vi "test.vi"() -> ()   [LabVIEW 2016]
uses:
  <vilib>/Platform/TimedLoop/XDataNode/timing_clust.ctl
  <vilib>/Platform/TimedLoop/XDataNode/nitl_modes.ctl
  <vilib>/Platform/TimedLoop/XDataNode/wakeup.ctl
  <vilib>/FPGAPlugInAG/roboRIO/niLvFpga_Open_roboRIO.vi
  <vilib>/rvi/interface/common/dynamic/niFpgaDynamicAddResources.vi
  <vilib>/FPGAPlugInAG/Dynamic/niLvFpga_Reset_Dynamic.vi
  <vilib>/FPGAPlugInAG/Dynamic/niLvFpga_Run_Dynamic.vi
  <vilib>/Utility/error.llb/Error Cluster From Error Code.vi
  <vilib>/rvi/errors/niLvFpgaAdjustHostInterfaceError.vi
  <vilib>/FPGAPlugInAG/Dynamic/niLvFpga_Abort_Dynamic.vi
  <vilib>/FPGAPlugInAG/Dynamic/niLvFpga_Close_Dynamic.vi
  <vilib>/rvi/interface/nirviOpenFPGA/nirviOpenFPGA.xnode
  FPGA Bitfiles/AutoBikeProject_FPGATarget_AutoBikeFPGA_EwzLm8KNttI.lvbitx
  <vilib>/rvi/interface/nirviMethod/nirviMethod.xnode
  <vilib>/platform/TimedLoop/XDataNode/XDataNode.xnode
  <vilib>/rvi/interface/nirviReadWriteControl/nirviReadWriteControl.xnode
  <vilib>/rvi/interface/nirviCloseFPGA/nirviCloseFPGA.xnode
  NiFpgaLv.dll
  <vilib>/rvi/interface/Simulation/niFpgaSimulationCallBeginRW.vi
  <vilib>/Platform/TimedLoop/XDataNode/XDNodeRunTimeDep.lvlib
panel:
  out "x+y":i32
  out "Finished Late? [i-1]":bool
  out "error out":errorcluster
  in  "Boolean":bool
  out "Current velocity":sgl(graph)
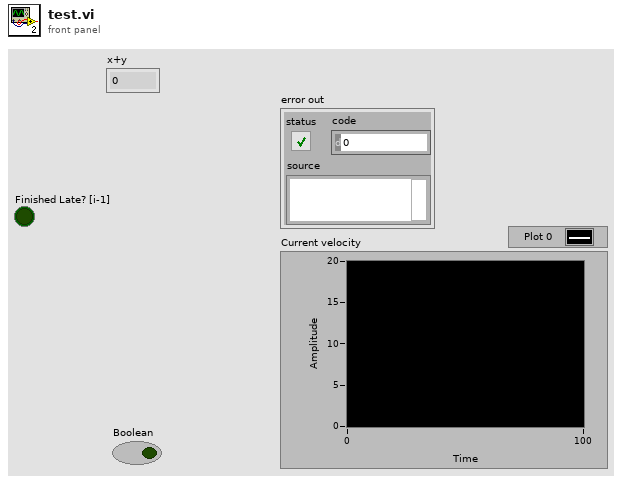
[diagram p1: front panel]
types:
  T1 = enum16{"open", "open or create", "create or replace", "create", "open (read-only)"}
  T2 = typedef "XDNodeRunTimeDep.lvlib/timing_clust.ctl" = cluster{"Expected End [f-1]":u64, "Actual End [f-1]":u64, "Finished Late? [f-1]":bool, "Expected End [i-1]":u64, "Actual End [i-1]":u64, "Finished Late? [i-1]":bool, "Expected Start [i]":u64, "Actual Start [i]":u64, "Expected Start [f]":u64, "Actual Start [f]":u64, "Source Name":string, "Structure Name":string, "Period":i64, "Deadline":i64, "Offset":i64, "Start":i64, "Priority":i32, "Timeout":i32, "Mode":T3, "Wakeup Reason":T4, "Error":errorcluster, "Source Type":string, "Secondary Source Type":string, "Global End Time":u64, "Global Start Time":u64, "Frame Duration":u64, "Iteration Duration":u64, "Assigned CPU":i32, "I/O Scan Engine Mode":u32}
  T3 = typedef "XDNodeRunTimeDep.lvlib/nitl_modes.ctl" = enum32{"No Change", "Process missed periods, maintain original phase", "Discard missed periods, maintain original phase", "Process missed periods, ignore original phase", "Discard missed periods, ignore original phase"}
  T4 = typedef "XDNodeRunTimeDep.lvlib/wakeup.ctl" = enum32{"Normal", "Aborted", "Asynchronous wakeup", "Timing source error", "Timed loop error", "Timeout"}
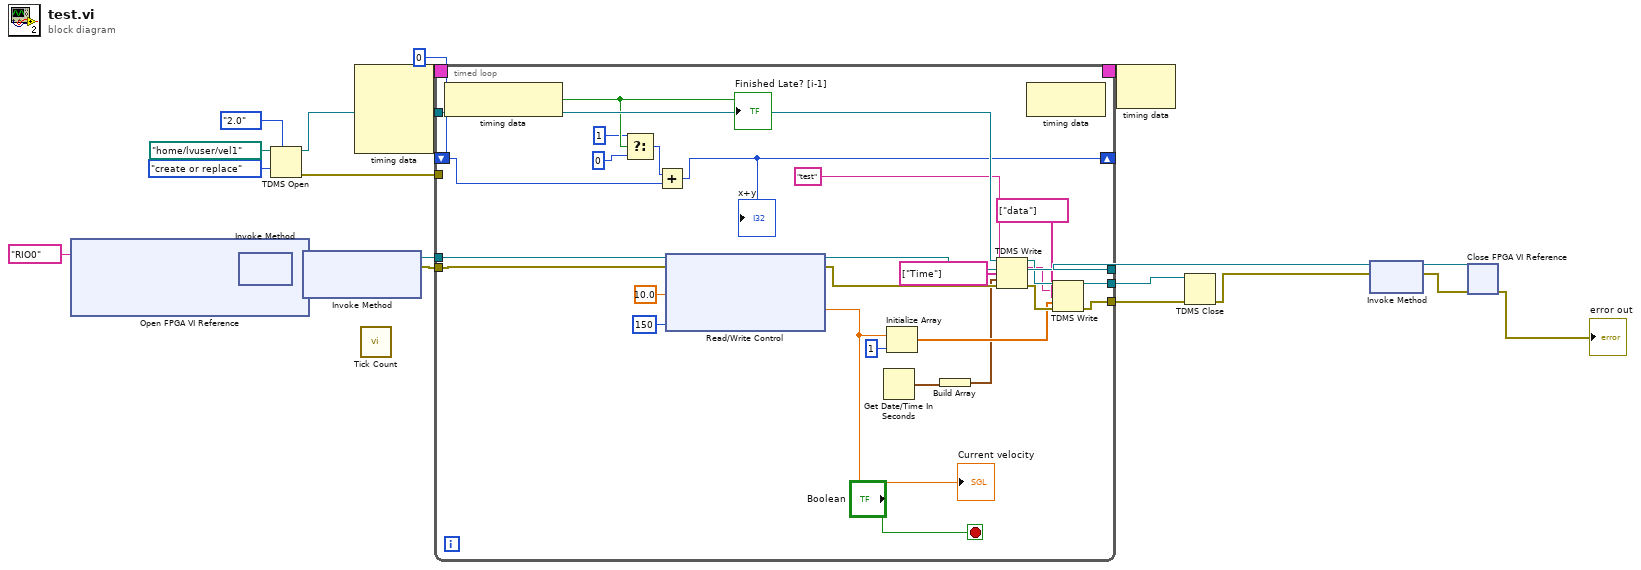
[diagram p0: block diagram]
diagram:
  n1 = xnode "Open FPGA VI Reference"("resource name"=tag "RIO0") -> ("FPGA VI Reference Out"=w22:refnum<k20>, "error out"=w21:errorcluster)  [unwired: 1 in]
  n2 = xnode "Invoke Method"("FPGA VI Reference In"=w22, "error in"=w21) -> ("FPGA VI Reference Out"=w20:refnum<k20>, "error out"=w19:errorcluster)
  n3 = TDMS Open(7:enum16{"1.0", "2.0"}."2.0" ("file format version (2.0)"), 10:T1."create or replace" ("operation (0:open)"), 11:path "/home/lvuser/vel1" ("file path")) -> (0:w8:errorcluster, 3:w9:refnum<k34>)  [unwired: 4 in]
  n4 = xnode "Invoke Method"("FPGA VI Reference In"=w20, "error in"=w19) -> ("FPGA VI Reference Out"=w18:refnum<k20>, "error out"=w17:errorcluster)  [unwired: 1 in]
  n5 = node-c288() -> (w3:T2)  [unwired: 4 in]
  n6 = call "Tick Count"() -> ()  [unwired: 1 out]
  n7 = timed-loop {
    tunnel: w18 -> [w48]
    tunnel: w17 -> [w47]
    tunnel: [w44] -> w16
    tunnel: w9 -> [w38]
    tunnel: w8 -> [_]
    tunnel: [w39] -> w7
    tunnel: [w36] -> w6
    timing: w3 -> [_]
    timing-out: [_] -> w2
    shift-right: [w24] -> _
    shift-left: 0 -> [w23]
    stop <- "Boolean" stop-if-true
    n8 = node-c288() -> (w28:bool)  [unwired: 1 in]
    "Finished Late? [i-1]" <- w28
    n9 = Select(t=1, s=w28, f=0) -> (s? t:f=w25:i32)
    n10 = Add(x=w25, y=w23) -> (x+y=w24:i32)
    "x+y" <- w24
    n11 = xnode "Read/Write Control"("FPGA VI Reference In"=w48, "error in"=w47, "Reference velocity in km/h"=sgl 10.0, "Count(uSec)"=u32 150) -> ("FPGA VI Reference Out"=w44:refnum<k20>, "error out"=w41:errorcluster, "Current velocity"=w42:sgl)  [unwired: 1 out]
    "Current velocity" <- w42
    n12 = Get Date/Time In Seconds() -> (seconds since 1Jan1904=w29:timestamp)
    n13 = Initialize Array(w42, 1 ("dimension size")) -> (w35:sgl[])
    n14 = Build Array(w29) -> (w30:timestamp[])
    n15 = TDMS Write(0:w38, 5:"test" ("group name in (Untitled)"), 7:string[] ["Time"] ("channel name(s) in (Untitled)"), 9:w30, 11:w41) -> (4:w40:refnum<k34>, 6:w31:string, 15:w37:errorcluster)  [unwired: 1 in, 1 out]
    n16 = node-c288() -> ()  [unwired: 1 in, 1 out]
    n17 = TDMS Write(0:w40, 5:w31, 7:string[] ["data"] ("channel name(s) in (Untitled)"), 9:w35, 11:w37) -> (4:w39:refnum<k34>, 15:w36:errorcluster)  [unwired: 1 in, 2 out]
  }
  n18 = node-c288(w2) -> ()  [unwired: 1 out]
  n19 = TDMS Close(8:w6, 11:w7) -> (0:w5:errorcluster)  [unwired: 1 out]
  n20 = xnode "Invoke Method"("FPGA VI Reference In"=w16, "error in"=w5) -> ("FPGA VI Reference Out"=w15:refnum<k20>, "error out"=w14:errorcluster)
  n21 = xnode "Close FPGA VI Reference"("FPGA VI Reference In"=w15, "error in"=w14) -> ("error out"=→"error out":errorcluster)
